vi "CMN_AnalizeFileTpl.vi"(10 "line string":string, 11 "number of Extensions":u16) -> (3 "Extensions":i32[][](array[numeric]))   [LabVIEW 2016]
panel:
  out "size(s)":i32
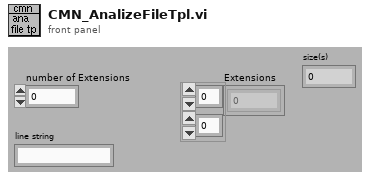
[diagram p1: front panel]
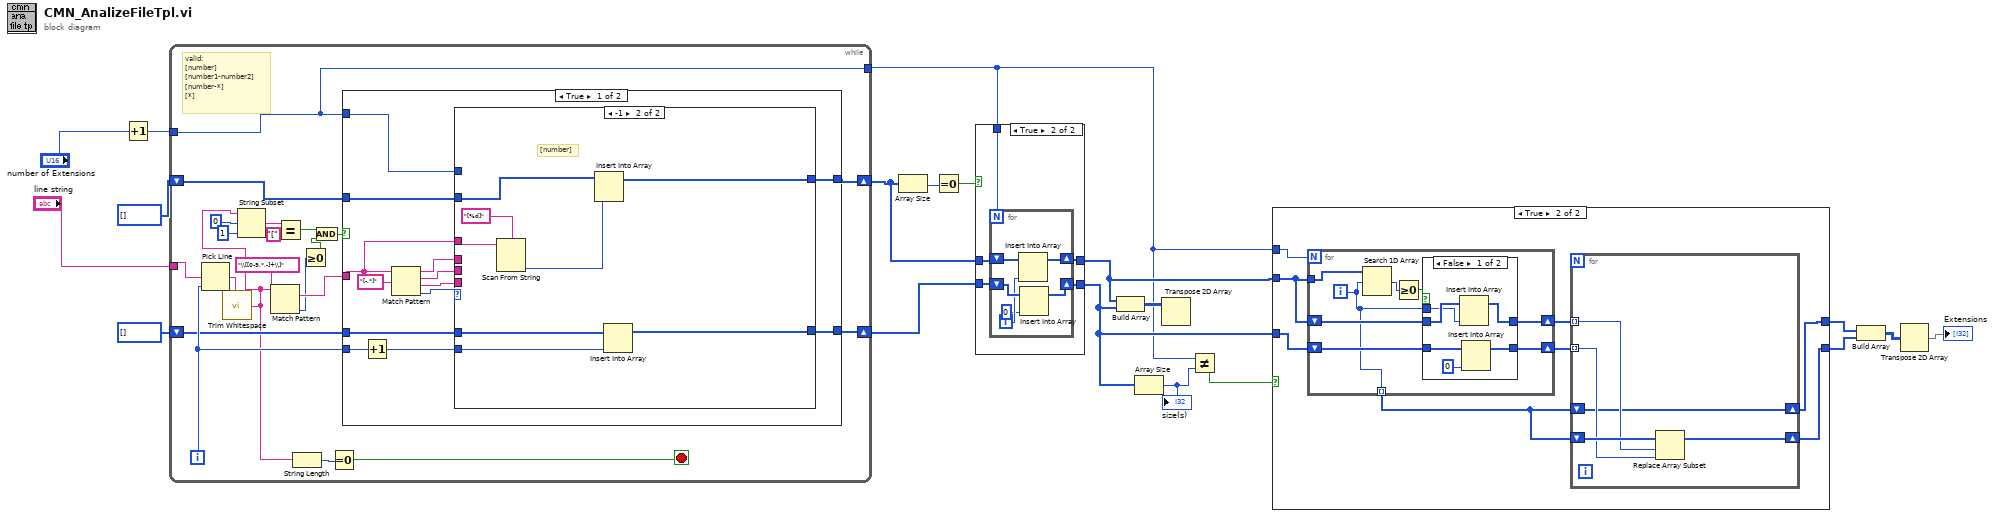
[diagram p0: block diagram]
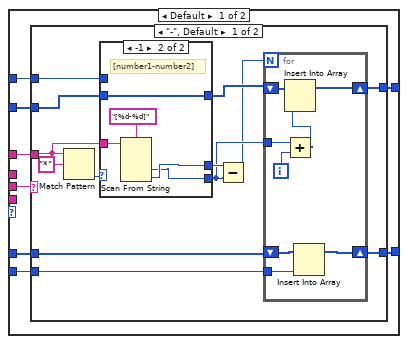
[diagram p4: hidden frame]
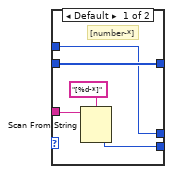
[diagram p5: hidden frame]
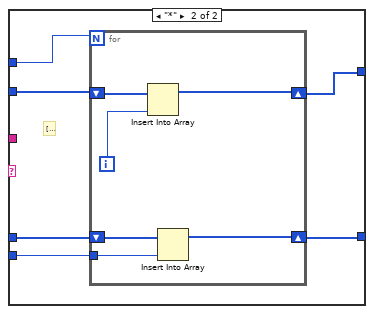
[diagram p6: hidden frame]
diagram:
  n1 = Increment(x="number of Extensions") -> (x+1=w10:u16)
  n2 = while {
    tunnel: [w29] -> w5
    shift-left: i32[] [] -> [w30]
    shift-right: [w31] -> w13
    tunnel: w10 -> [w29]
    shift-left: i32[] [] -> [w34]
    shift-right: [w35] -> w12
    tunnel: "line string" -> [w33]
    i -> [w32]
    stop <- w37 stop-if-true
    # "valid:\n[number]\n[number1-number2]\n[number-*]\n[*]"
    n3 = Pick Line(multi-line string=w33, line index=w32) -> (output string=w39:string)  [unwired: 1 out]
    n4 = call <vilib>:"Trim Whitespace.vi"("string"=w39) -> ("trimmed string"=w24:string)  [unwired: 1 in]
    n5 = String Subset(string=w24, offset (0)=0, length (rest)=1 ("length (rest)")) -> (substring=w27:string)
    n6 = Match Pattern(string=w24, regular expression="\\[[0-9,*,-]+\\]") -> (match substring=w36:string, offset past match=w22:i32)  [unwired: 3 out]
    n7 = Equal?(x=w27, y="[") -> (x = y?=w23:bool)
    n8 = String Length(string=w24) -> (length=w38:i32)
    n9 = Greater Or Equal To 0?(x=w22) -> (x >= 0?=w21:bool)
    n10 = And(x=w23, y=w21) -> (x .and. y?=w20:bool)
    n11 = Equal To 0?(x=w38) -> (x = 0?=w37:bool)
    n12 = case shown="True" w20 {
      tunnel: w36 -> [w51 _]
      tunnel: [w50 w114] -> w35
      tunnel: w34 -> [w49 w114]
      tunnel: w29 -> [w45 _]
      tunnel: w32 -> [w44 _]
      tunnel: [w43 w113] -> w31
      tunnel: w30 -> [w42 w113]
      frame True {
        n13 = Increment(x=w44) -> (x+1=w41:i32)
        n14 = Match Pattern(string=w51, regular expression="[-,*]") -> (before substring=w48:string, match substring=w46:string, after substring=w47:string, offset past match=w52:i32)  [unwired: 1 out]
        n15 = case shown="-1" w52 {
          tunnel: w51 -> [w60 w110]
          tunnel: [w57 w112] -> w50
          tunnel: w49 -> [w59 w111]
          tunnel: w48 -> [_ _]
          tunnel: w47 -> [_ _]
          tunnel: w46 -> [w61 _]
          tunnel: w45 -> [w58 _]
          tunnel: w41 -> [w55 w107]
          tunnel: [w54 w106] -> w43
          tunnel: w42 -> [w56 w105]
          frame Default {
            n16 = case shown="\"-\", Default" w61 {
              tunnel: w60 -> [w72 _]
              tunnel: w59 -> [w71 w98]
              tunnel: w58 -> [w70 w93]
              tunnel: [w66 w97] -> w57
              tunnel: w56 -> [w65 w95]
              tunnel: w55 -> [w63 w96]
              tunnel: [w64 w94] -> w54
              frame "-", Default {
                n17 = Match Pattern(string=w72, regular expression="*") -> (offset past match=w73:i32)  [unwired: 4 out]
                n18 = case shown="-1" w73 {
                  tunnel: w72 -> [w87 w91]
                  tunnel: w71 -> [w85 w88]
                  tunnel: w70 -> [w83 _]
                  tunnel: [w83 w90] -> w69
                  tunnel: [w84 w89] -> w68
                  tunnel: [w85 w88] -> w67
                  frame Default {
                    # "[number-*]"
                    n19 = Scan From String(format string="[%d-*]" ("Format String"), input string=w87) -> (output 1=w84:i32)  [unwired: 2 in, 4 out]
                  }
                  frame -1 {
                    # "[number1-number2]"
                    n20 = Scan From String(format string="[%d-%d]" ("Format String"), input string=w91) -> (output 1=w89:i32, output 2=w90:i32)  [unwired: 2 in, 5 out]
                  }
                }
                n21 = Subtract(x=w69, y=w68) -> (x-y=w62:i32)
                n22 = for {
                  N: w62 -> [_]
                  shift-right: [w80] -> w66
                  shift-left: w67 -> [w78]
                  tunnel: w68 -> [w79]
                  shift-right: [w76] -> w64
                  shift-left: w65 -> [w77]
                  tunnel: w63 -> [w75]
                  i -> [w82]
                  n23 = Add(x=w79, y=w82) -> (x+y=w81:i32)
                  n24 = Insert Into Array(array=w78, new element=w81) -> (w80:i32[])  [unwired: 1 in]
                  n25 = Insert Into Array(array=w77, new element=w75) -> (w76:i32[])  [unwired: 1 in]
                }
              }
              frame "*" {
                # "[*]"
                n26 = for {
                  N: w93 -> [_]
                  shift-right: [w99] -> w97
                  shift-left: w98 -> [w104]
                  tunnel: w96 -> [w102]
                  shift-right: [w100] -> w94
                  shift-left: w95 -> [w101]
                  i -> [w103]
                  n27 = Insert Into Array(array=w104, new element=w103) -> (w99:i32[])  [unwired: 1 in]
                  n28 = Insert Into Array(array=w101, new element=w102) -> (w100:i32[])  [unwired: 1 in]
                }
              }
            }
          }
          frame -1 {
            # "[number]"
            n29 = Scan From String(format string="[%d]" ("Format String"), input string=w110) -> (output 1=w108:i32)  [unwired: 2 in, 4 out]
            n30 = Insert Into Array(array=w111, new element=w108) -> (w112:i32[])  [unwired: 1 in]
            n31 = Insert Into Array(array=w105, new element=w107) -> (w106:i32[])  [unwired: 1 in]
          }
        }
      }
      frame False {
      }
    }
  }
  n32 = Array Size(array=w12) -> (size(s)=w15:i32)
  n33 = Equal To 0?(x=w15) -> (x = 0?=w14:bool)
  n34 = case shown="True" w14 {
    tunnel: w13 -> [w115 w120]
    tunnel: w12 -> [w116 w121]
    tunnel: [w116 w117] -> w6
    tunnel: w5 -> [_ w119]
    tunnel: [w115 w118] -> w7
    frame False {
    }
    frame True {
      n35 = for {
        N: w119 -> [_]
        shift-right: [w125] -> w117
        shift-left: w121 -> [w126]
        shift-right: [w124] -> w118
        shift-left: w120 -> [w127]
        i -> [w123]
        n36 = Insert Into Array(array=w126, new element=w123) -> (w125:i32[])  [unwired: 1 in]
        n37 = Insert Into Array(array=w127, new element=0 ("New Element/Subarray")) -> (w124:i32[])  [unwired: 1 in]
      }
    }
  }
  n38 = Build Array(w6, w7) -> (w16:i32[][])
  n39 = Array Size(array=w7) -> (size(s)=w9:i32)
  "size(s)" <- w9
  n40 = Transpose 2D Array(2D array=w16) -> ()  [unwired: 1 out]
  n41 = Not Equal?(x=w5, y=w9) -> (x != y?=w8:bool)
  n42 = case shown="True" w8 {
    tunnel: w7 -> [w128 w136]
    tunnel: w6 -> [w129 w137]
    tunnel: w5 -> [_ w135]
    tunnel: [w129 w131] -> w4
    tunnel: [w128 w130] -> w3
    frame False {
    }
    frame True {
      n43 = for {
        N: w135 -> [_]
        tunnel: w137 -> [w144]
        shift-right: [w147] -> w132
        shift-left: w137 -> [w148]
        shift-right: [w145] -> w134
        shift-left: w136 -> [w146]
        tunnel: [w143] -> w133 mode=indexing
        i -> [w143]
        n44 = Search 1D Array(1D array=w144, element=w143) -> (index of element=w150:i32)  [unwired: 1 out]
        n45 = Greater Or Equal To 0?(x=w150) -> (x >= 0?=w149:bool)
        n46 = case shown="False" w149 {
          tunnel: w148 -> [w156 w158]
          tunnel: [w155 w158] -> w147
          tunnel: w146 -> [w153 w157]
          tunnel: [w152 w157] -> w145
          tunnel: w143 -> [w154 _]
          frame False {
            n47 = Insert Into Array(array=w156, new element=w154) -> (w155:i32[])  [unwired: 1 in]
            n48 = Insert Into Array(array=w153, new element=0 ("new element/subarray")) -> (w152:i32[])  [unwired: 1 in]
          }
          frame True {
          }
        }
      }
      n49 = for {
        shift-right: [w139] -> w131
        shift-left: w133 -> [w139]
        tunnel: w134 -> [w140] mode=indexing
        shift-right: [w138] -> w130
        shift-left: w133 -> [w142]
        tunnel: w132 -> [w141] mode=indexing
        n50 = Replace Array Subset(array=w142, new element=w140, index=w141) -> (w138:i32[])
      }
    }
  }
  n51 = Build Array(w4, w3) -> (w2:i32[][])
  n52 = Transpose 2D Array(2D array=w2) -> (transposed array=→"Extensions":i32[][])
